vi "Close to SFTP.vi"(8 "Error In":errorcluster, 11 "SFTP File":refnum<class "SFTP File.lvclass">) -> (0 "Error Out":errorcluster, 2 "Remote Path":string, 3 "SFTP":refnum<class "SFTP.lvclass">)   [LabVIEW 2018, in "Toolkit.lvlib" / "SFTP File.lvclass"]
doc: "Destroys this SFTP File object and returns the SFTP object used to originally create it."
uses:
  SFTP File.lvclass
  SFTP/SFTP.lvclass
  SFTP File.lvclass/SFTP File.ctl
  SFTP/SFTP.lvclass/SFTP.ctl
  Session/Session.lvclass/Session.ctl
  SSH/SSH.lvclass/SSH.ctl
  Toolkit.lvlib
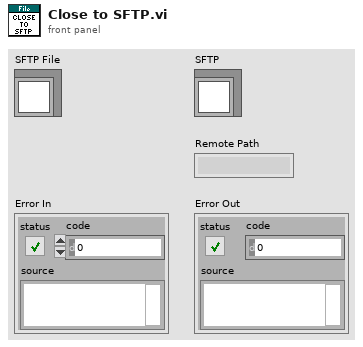
[diagram p1: front panel]
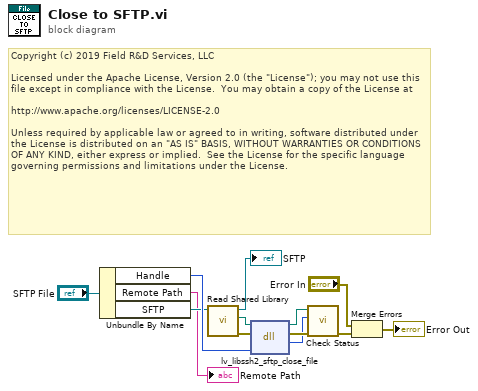
[diagram p0: block diagram]
diagram:
  # "Copyright (c) 2019 Field R&D Services, LLC\n\nLicensed under the Apache License, Version 2.0 (the \"License\"); you may not use this file except in compliance with the License.  You may obtain a copy of the License at\n\nhttp://www.apache.org/licenses/LICENSE-2.0\n\nUnless required by applicable law or agreed to in writing, software distributed under the License is distributed on an \"AS IS\" BASIS, WITHOUT WARRANTIES OR CONDITIONS OF ANY KIND, either express or implied.  See the License for the specific language governing permissions and limitations under the License."
  n1 = Unbundle By Name("SFTP File") -> ("Handle"=w11:u64, "Remote Path"=→"Remote Path":string, "SFTP"=w5:refnum<class "SFTP.lvclass">)
  n2 = call "Read Shared Library.vi"("SFTP In"=w5) -> ("Erorr Out"=w2:errorcluster, "libssh2lv Shared Library"=w3:path, "SFTP Out"=→"SFTP":refnum<class "SFTP.lvclass">)  [unwired: 8 in]
  n3 = dll-call lib="D:/Users/cfield/Code/Field R&D Services/SSH/LV-LIBSSH2/LabVIEW/trunk/src/Toolkit/Support/lv-libssh2.dll" fn="lv_libssh2_sftp_close_file"(path in=w3, error in=w2, "handle"=w11) -> (path out=w9:path, error out=w10:errorcluster, "status"=w7:i32)  [unwired: 2 in]
  n4 = call "Check Status.vi"("Error In"=w10, "Status"=w7, "libssh2lv Shared Library In"=w9) -> ("Error Out"=w8:errorcluster)  [unwired: 7 in, 1 out]
  n5 = Merge Errors("Error In", w8) -> (→"Error Out":errorcluster)
